vi "Untitled 0.vi"() -> ()   [LabVIEW 2016]
uses:
  <vilib>/picture/picture.llb/Draw True-Color Pixmap.vi
  <vilib>/Analysis/Matrix/Numeric/Conversions/Array To Matrix - RA2.vi
  <vilib>/imath/engines/lvmath2/RunTimeEngine/Managers/WorkSpace/UID Generator.vi
  <vilib>/Analysis/Matrix/Numeric/Conversions/Matrix To Array - RM.vi
  <vilib>/imath/engines/lvmath2/RunTimeEngine/BuiltInFunctions/rotate90/NIMS_rotate90.vi
  <instcachedir>/0/NIMS_rotate90_7DC1660D109944E092D2EB6E3185A1B6.lvgen/NIMS_rotate90_7DC1660D109944E092D2EB6E3185A1B6_004.vi
  <vilib>/imath/engines/lvmath2/RunTimeEngine/RunTimeType/NIMS_RunTimeType_From StrictType (excl LVString).vi
  <instcachedir>/0/NIMS_RunTimeType_From StrictType (excl LVString)_BBF44FB49F834B71AF7A14CCEDF8BECD.lvgen/NIMS_RunTimeType_From StrictType (excl LVString)_BBF44FB49F834B71AF7A14CCEDF8BECD_000.vi
  <vilib>/imath/engines/lvmath2/RunTimeEngine/LocalVariableDefStatement/MC_LocalVariableDefStatement_Display.vi
  <vilib>/imath/engines/lvmath2/RunTimeEngine/RangeToken/NIMS_Range_R2 - Integer.vi
  <instcachedir>/0/NIMS_Range_R2 - Integer_89B873E74E6E489885E44F751DD9C6BF.lvgen/NIMS_Range_R2 - Integer_89B873E74E6E489885E44F751DD9C6BF_000.vi
  <vilib>/imath/engines/lvmath2/RunTimeEngine/CommandStatement/MC_CommandStatement_break.vi
  <vilib>/imath/engines/lvmath2/RunTimeEngine/RangeToken/NIMS_Range.vi
  <instcachedir>/0/NIMS_Range_A7C094595B484CA7AF10685B02D808ED.lvgen/NIMS_Range_A7C094595B484CA7AF10685B02D808ED_000.vi
  <vilib>/imath/engines/lvmath2/RunTimeSupport/NIMS_Error if Not Equal.vi
  <instcachedir>/0/NIMS_Error if Not Equal_43252A79AD05436189442EC0C5E5AB8A.lvgen/NIMS_Error if Not Equal_43252A79AD05436189442EC0C5E5AB8A_001.vi
  <vilib>/imath/engines/lvmath2/RunTimeEngine/IndexRead/NIMS M(V,S).vi
  <instcachedir>/0/NIMS M(V,S)_4A7282EC9BD94252BB5D44AC841A97D6.lvgen/NIMS M(V,S)_4A7282EC9BD94252BB5D44AC841A97D6_001.vi
  <vilib>/imath/engines/lvmath2/RunTimeEngine/IndexReplace/NIMS M(V,S)=V.vi
  <instcachedir>/0/NIMS M(V,S)=V_F75C9F1BFECF4A57AE59A9C096BE65FD.lvgen/NIMS M(V,S)=V_F75C9F1BFECF4A57AE59A9C096BE65FD_001.vi
  <vilib>/imath/engines/lvmath2/RunTimeEngine/ErrorHandling/NIMS_Create Error From Enums.vi
  <vilib>/imath/engines/lvmath2/RunTimeEngine/Managers/SymbolTable/Clear UID.vi
  <vilib>/imath/engines/lvmath2/RunTimeEngine/NodeEndStatement/NIMS_NodeEndStatement_Output.vi
  <instcachedir>/0/NIMS_NodeEndStatement_Output_53EC0D466D134D7ABD903AC30B43404B.lvgen/NIMS_NodeEndStatement_Output_53EC0D466D134D7ABD903AC30B43404B_002.vi
  <vilib>/imath/engines/lvmath2/RunTimeEngine/ErrorHandling/NIMS_Finalize Error.vi
  <vilib>/imath/engines/lvmath2/RunTimeEngine/IndexRead/NIMS M(S,V).vi
  <instcachedir>/0/NIMS M(S,V)_5C1965D37F59432CA0E9661793EAFE90.lvgen/NIMS M(S,V)_5C1965D37F59432CA0E9661793EAFE90_001.vi
  <vilib>/imath/engines/lvmath2/RunTimeEngine/IndexReplace/NIMS M(S,V)=V.vi
  <instcachedir>/0/NIMS M(S,V)=V_00A569AEF20C4D858392F22F057607EC.lvgen/NIMS M(S,V)=V_00A569AEF20C4D858392F22F057607EC_001.vi
  <vilib>/imath/engines/lvmath2/RunTimeEngine/BuiltInFunctions/round/NIMS_round(DBL-S).vi
  <vilib>/imath/engines/lvmath2/RunTimeEngine/BuiltInFunctions/zeros/NIMS_M=zeros(I32,I32).vi
  <vilib>/imathl/engines/lvmath/Functions/Error Handling/Create Error.vi
  <vilib>/imath/engines/lvmath2/RunTimeEngine/RangeToken/NIMS_Range_R2 - Float.vi
  <instcachedir>/0/NIMS_Range_R2 - Float_590A1087448447AEB7F770FC082D3801.lvgen/NIMS_Range_R2 - Float_590A1087448447AEB7F770FC082D3801_000.vi
  <instcachedir>/0/NIMS_Error if Not Equal_43252A79AD05436189442EC0C5E5AB8A.lvgen/NIMS_Error if Not Equal_43252A79AD05436189442EC0C5E5AB8A_000.vi
  <vilib>/imath/engines/lvmath2/RunTimeEngine/IndexRead/NIMS M(S,$).vi
  <instcachedir>/0/NIMS M(S,$)_F24F360562DE41D8BE234322A2E15C65.lvgen/NIMS M(S,$)_F24F360562DE41D8BE234322A2E15C65_002.vi
  <vilib>/imath/engines/lvmath2/RunTimeEngine/IndexReplace/NIMS M(S,$)=V.vi
  <instcachedir>/0/NIMS M(S,$)=V_BCCFA522A894489B8FA760383D74A164.lvgen/NIMS M(S,$)=V_BCCFA522A894489B8FA760383D74A164_001.vi
  <vilib>/imath/engines/lvmath2/RunTimeEngine/IndexRead/NIMS M($,S).vi
  <instcachedir>/0/NIMS M($,S)_3E5749BBB62E49528D4765A77F1F6D98.lvgen/NIMS M($,S)_3E5749BBB62E49528D4765A77F1F6D98_002.vi
  <vilib>/imath/engines/lvmath2/RunTimeEngine/IndexReplace/NIMS M($,S)=V.vi
  <instcachedir>/0/NIMS M($,S)=V_EEA74323A7E5479BB387BE0F93352290.lvgen/NIMS M($,S)=V_EEA74323A7E5479BB387BE0F93352290_002.vi
  <instcachedir>/0/NIMS_NodeEndStatement_Output_53EC0D466D134D7ABD903AC30B43404B.lvgen/NIMS_NodeEndStatement_Output_53EC0D466D134D7ABD903AC30B43404B_010.vi
  <vilib>/imath/engines/lvmath2/RunTimeEngine/BuiltInFunctions/rand/NIMS_rand(I32,I32).vi
  <vilib>/imath/engines/lvmath2/RunTimeEngine/ErrorHandling/NIMS_Error From Error Code.vi
  <vilib>/imath/engines/lvmath2/RunTimeEngine/ArithmeticOperatorToken/NIMS_ArithmeticOperator_minus.vi
  <instcachedir>/0/NIMS_ArithmeticOperator_minus_E3B65B1D26A44BB184AFDC5B3F458E3D.lvgen/NIMS_ArithmeticOperator_minus_E3B65B1D26A44BB184AFDC5B3F458E3D_003.vi
  <instcachedir>/0/NIMS M(S,$)=V_BCCFA522A894489B8FA760383D74A164.lvgen/NIMS M(S,$)=V_BCCFA522A894489B8FA760383D74A164_000.vi
  <vilib>/imath/engines/lvmath2/RunTimeEngine/ArithmeticOperatorToken/NIMS_ArithmeticOperator_plus.vi
  <instcachedir>/0/NIMS_ArithmeticOperator_plus_0120E0498A0F4B4B9BDCAC2554767A4E.lvgen/NIMS_ArithmeticOperator_plus_0120E0498A0F4B4B9BDCAC2554767A4E_004.vi
  <instcachedir>/0/NIMS M($,S)=V_EEA74323A7E5479BB387BE0F93352290.lvgen/NIMS M($,S)=V_EEA74323A7E5479BB387BE0F93352290_001.vi
  <instcachedir>/0/NIMS_ArithmeticOperator_plus_0120E0498A0F4B4B9BDCAC2554767A4E.lvgen/NIMS_ArithmeticOperator_plus_0120E0498A0F4B4B9BDCAC2554767A4E_003.vi
  <vilib>/Analysis/Matrix/NI_Matrix.lvlib
  <vilib>/imath/engines/lvmath2/RunTimeEngine/Managers/SymbolTable/NIMS_WorkSpace.lvlib
panel:
  in  "Cluster":T1 {"y 2" scale=0.0..4.0; "Meter" scale=-360.0..360.0 scale format="%#_3g"; "y" scale=-500.0..500.0; "x" scale=-500.0..500.0}
  out "new picture 2":picture
  in  "Enum":T2(ring)
  out "new picture":picture
  in  "File Path Control":path
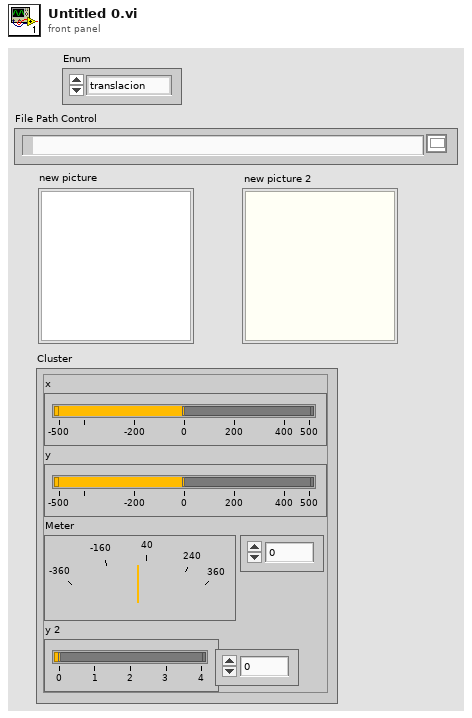
[diagram p1: front panel]
types:
  T1 = cluster{"x":dbl, "y":dbl, "Meter":dbl, "y 2":i64}
  T2 = enum16{"translacion", "giro", "extraccion", "zoom", "giroH", "giroV"}
  T3 = typedef "imagedata.ctl" = cluster{"image type":i32, "image depth":i32, "image":u8[], "mask":u8[], "colors":u32[], "Rectangle":cluster{"left":i16, "top":i16, "right":i16, "bottom":i16}}
  T4 = cluster{"left":i16, "top":i16, "right":i16, "bottom":i16}
  T5 = typedef "NI_Matrix.lvlib/RealMatrix.ctl" = dbl[][]
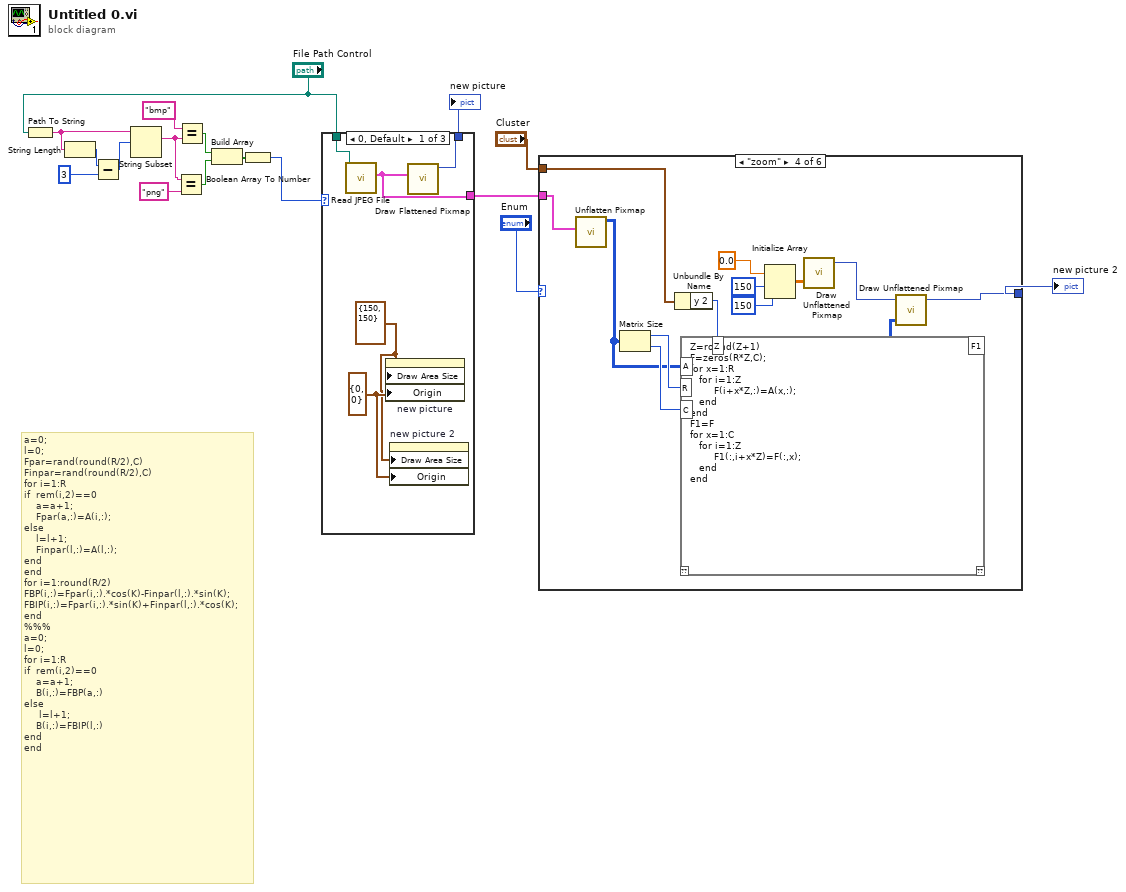
[diagram p0: block diagram]
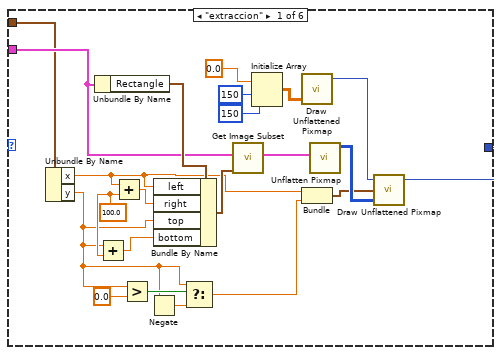
[diagram p2: hidden frame]
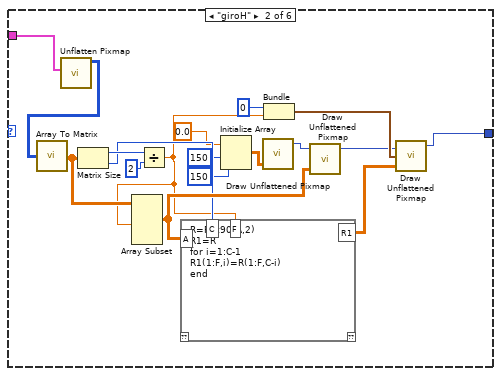
[diagram p3: hidden frame]
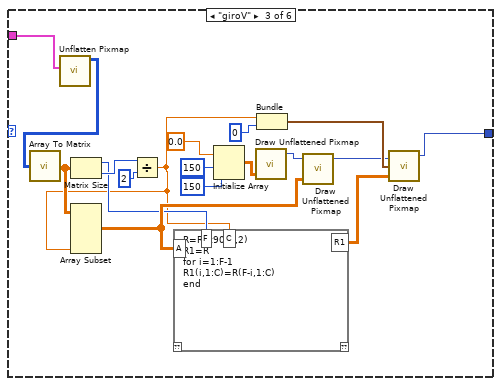
[diagram p4: hidden frame]
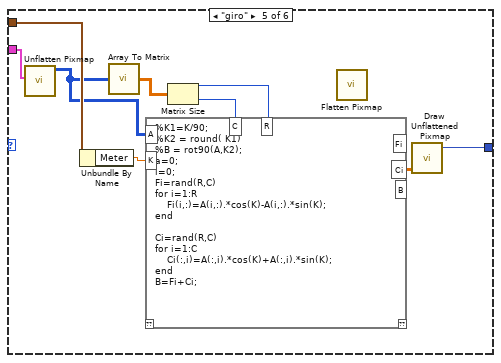
[diagram p5: hidden frame]
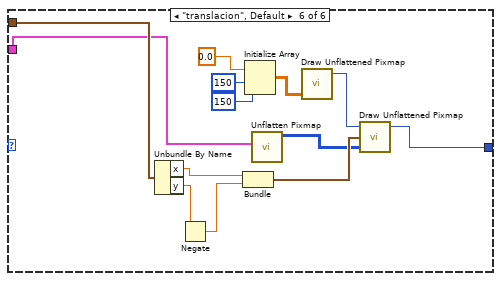
[diagram p6: hidden frame]
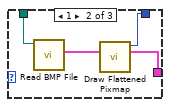
[diagram p7: hidden frame]
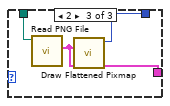
[diagram p8: hidden frame]
diagram:
  # "a=0;\nl=0;\nFpar=rand(round(R/2),C)\nFinpar=rand(round(R/2),C)\nfor i=1:R\nif  rem(i,2)==0\n    a=a+1;\n    Fpar(a,:)=A(i,:);\nelse\n    l=l+1;\n    Finpar(l,:)=A(l,:);\nend\nend\nfor i=1:round(R/2)\nFBP(i,:)=Fpar(i,:).*cos(K)-Finpar(l,:).*sin(K);\nFBIP(i,:)=Fpar(i,:).*sin(K)+Finpar(l,:).*cos(K);\nend\n%%%\na=0;\nl=0;\nfor i=1:R\nif  rem(i,2)==0\n    a=a+1;\n    B(i,:)=FBP(a,:)\nelse\n     l=l+1;\n    B(i,:)=FBIP(l,:)\nend \nend"
  n1 = Path To String(path="File Path Control") -> (string=w4:string)
  n2 = String Length(string=w4) -> (length=w17:i32)
  n3 = Subtract(x=w17, y=3) -> (x-y=w15:i32)
  n4 = String Subset(string=w4, offset (0)=w15) -> (substring=w5:string)  [unwired: 1 in]
  n5 = Equal?(x=w5, y="png" ("x")) -> (x = y?=w10:bool)
  n6 = Equal?(x="bmp", y=w5) -> (x = y?=w9:bool)
  n7 = Build Array(w9, w10) -> (w11:bool[])
  n8 = Boolean Array To Number(Boolean array=w11) -> (number=w12:u32)
  n9 = case shown="0, Default" w12 {
    tunnel: [w22 w25 w27] -> w3
    tunnel: "File Path Control" -> [w21 w24 w28]
    tunnel: [w20 w23 w26] -> w2
    frame 0, Default {
      w19 = cluster{"Horizontal":i16, "Vertical":i16} {"Horizontal"=0, "Vertical"=0} ("Origin")
      w18 = cluster{"Width":u32, "Height":u32} {"Width"=150, "Height"=150} ("Caption.Size")
      n10 = call <vilib>:"Read JPEG File.vi"("path to JPEG file"=w21) -> ("image data"=w20:T3)  [unwired: 8 in, 2 out]
      n11 = property on="new picture" class="Pict"("Draw Area Size"=w18, "Origin"=w19) -> ()  [unwired: 2 in, 2 out]
      n12 = property on="new picture 2" class="Pict"("Draw Area Size"=w18, "Origin"=w19) -> ()  [unwired: 2 in, 2 out]
      n13 = call <vilib>:"Draw Flattened Pixmap.vi"("image data"=w20) -> ("new picture"=w22:picture)  [unwired: 8 in]
    }
    frame 1 {
      n14 = call <vilib>:"Read BMP File.vi"("path to BMP file"=w24) -> ("image data"=w23:T3)  [unwired: 8 in, 2 out]
      n15 = call <vilib>:"Draw Flattened Pixmap.vi"("image data"=w23) -> ("new picture"=w25:picture)  [unwired: 8 in]
    }
    frame 2 {
      n16 = call <vilib>:"Read PNG File.vi"("path to PNG file"=w28) -> ("image data"=w26:T3)  [unwired: 8 in, 2 out]
      n17 = call <vilib>:"Draw Flattened Pixmap.vi"("image data"=w26) -> ("new picture"=w27:picture)  [unwired: 8 in]
    }
  }
  "new picture" <- w3
  n18 = case shown="\"zoom\"" "Enum" {
    tunnel: [w43 w67 w234 w394 w703 w970] -> w7
    tunnel: w2 -> [w48 w52 w219 w385 w698 w963]
    tunnel: "Cluster" -> [w42 _ _ w387 w700 w967]
    frame "extraccion" {
      w36 = 100.0 ("y")
      n19 = Unbundle By Name(w42) -> ("x"=w35:dbl, "y"=w29:dbl)
      n20 = Unbundle By Name(w48) -> ("Rectangle"=w50:T4)
      n21 = Add(x=w29, y=w36) -> (x+y=w47:dbl)
      n22 = Add(x=w35, y=w36) -> (x+y=w46:dbl)
      n23 = Greater?(x=w29, y=0.0) -> (0:w32:bool)
      n24 = Negate(x=w29) -> (-x=w30:dbl)
      n25 = Bundle By Name(cluster=w50, "left"=w35, "right"=w46, "top"=w29, "bottom"=w47) -> (w49:T4)
      n26 = Select(t=w29, s=w32, f=w30) -> (s? t:f=w31:dbl)
      n27 = call <vilib>:"Get Image Subset.vi"("subset rect"=w49, "image data"=w48) -> ("image subset"=w45:T3)  [unwired: 4 in, 1 out]
      n28 = Initialize Array(0.0 ("element"), 150 ("dimension size"), 150 ("dimension size")) -> (w38:dbl[][])
      n29 = call-poly <vilib>:"Draw Unflattened Pixmap.vi"("data (RGB format)"=w38) -> ("new picture"=w37:picture)  [unwired: 8 in]
      n30 = Bundle("x"=w35, "y"=w31) -> (w34:cluster{"x":dbl, "y":dbl})  [unwired: 1 in]
      n31 = call <vilib>:"Unflatten Pixmap.vi"("image data"=w45) -> ("24-bit pixmap"=w44:u32[][])  [unwired: 4 in, 6 out]
      n32 = call-poly <vilib>:"Draw Unflattened Pixmap.vi"("picture"=w37, "top left point(0, 0)"=w34, "data (RGB format)"=w44) -> ("new picture"=w43:picture)  [unwired: 6 in]
    }
    frame "giroH" {
      n33 = call <vilib>:"Unflatten Pixmap.vi"("image data"=w52) -> ("24-bit pixmap"=w51:u32[][])  [unwired: 4 in, 6 out]
      n34 = call-poly <vilib>:"Array To Matrix.vi"("Real 2D Array"=w51) -> ("Real Matrix"=w68:T5)
      n35 = Matrix Size(0:w68) -> (1:w61:i32, 2:w60:i32)
      n36 = Divide(x=w61, y=2) -> (x/y=w59:dbl)
      n37 = Array Subset(array=w68, length (row)=w59) -> (w63:T5)  [unwired: 3 in]
      n38 = mathscript code="R=Rot90(A,2)\nR1=R\nfor i=1:C-1\nR1(1:F,i)=R(1:F,C-i)\nend"("A"=w63, "C"=w60, "F"=w59) -> ("R1"=w58:dbl[][])  [unwired: 1 in, 1 out]
      n39 = Initialize Array(0.0 ("element"), 150 ("dimension size"), 150 ("dimension size")) -> (w54:dbl[][])
      n40 = call-poly <vilib>:"Draw Unflattened Pixmap.vi"("data (RGB format)"=w54) -> ("new picture"=w53:picture)  [unwired: 8 in]
      n41 = Bundle("y"=0, w59) -> (w64:cluster{"y":i32, dbl})  [unwired: 1 in]
      n42 = call-poly <vilib>:"Draw Unflattened Pixmap.vi"("picture"=w53, "data (RGB format)"=w63) -> ("new picture"=w62:picture)  [unwired: 7 in]
      n43 = call-poly <vilib>:"Draw Unflattened Pixmap.vi"("picture"=w62, "top left point(0, 0)"=w64, "data (RGB format)"=w58) -> ("new picture"=w67:picture)  [unwired: 6 in]
    }
    frame "giroV" {
      n44 = call <vilib>:"Unflatten Pixmap.vi"("image data"=w219) -> ("24-bit pixmap"=w218:u32[][])  [unwired: 4 in, 6 out]
      n45 = call-poly <vilib>:"Array To Matrix.vi"("Real 2D Array"=w218) -> ("Real Matrix"=w235:T5)
      n46 = Matrix Size(0:w235) -> (1:w222:i32, 2:w223:i32)
      n47 = Divide(x=w223, y=2) -> (x/y=w220:dbl)
      n48 = Array Subset(array=w235, length (col)=w220) -> (w231:T5)  [unwired: 3 in]
      n49 = mathscript code="R=Rot90(A,2)\nR1=R\nfor i=1:F-1\nR1(i,1:C)=R(F-i,1:C)\nend"("A"=w231, "F"=w222, "C"=w220) -> ("R1"=w229:dbl[][])  [unwired: 1 in, 1 out]
      n50 = Initialize Array(0.0 ("element"), 150 ("dimension size"), 150 ("dimension size")) -> (w225:dbl[][])
      n51 = call-poly <vilib>:"Draw Unflattened Pixmap.vi"("data (RGB format)"=w225) -> ("new picture"=w224:picture)  [unwired: 8 in]
      n52 = Bundle(w220, "y"=0) -> (w232:cluster{dbl, "y":i32})  [unwired: 1 in]
      n53 = call-poly <vilib>:"Draw Unflattened Pixmap.vi"("picture"=w224, "data (RGB format)"=w231) -> ("new picture"=w230:picture)  [unwired: 7 in]
      n54 = call-poly <vilib>:"Draw Unflattened Pixmap.vi"("picture"=w230, "top left point(0, 0)"=w232, "data (RGB format)"=w229) -> ("new picture"=w234:picture)  [unwired: 6 in]
    }
    frame "zoom" {
      n55 = call <vilib>:"Unflatten Pixmap.vi"("image data"=w385) -> ("24-bit pixmap"=w384:u32[][])  [unwired: 4 in, 6 out]
      n56 = Matrix Size(0:w384) -> (1:w396:i32, 2:w395:i32)
      n57 = Unbundle By Name(w387) -> ("y 2"=w386:i64)
      n58 = mathscript code="Z=round(Z+1)\nF=zeros(R*Z,C);\nfor x=1:R\n   for i=1:Z\n        F(i+x*Z,:)=A(x,:);\n   end\nend\nF1=F\nfor x=1:C\n   for i=1:Z\n        F1(:,i+x*Z)=F(:,x);\n   end\nend"("R"=w396, "C"=w395, "Z"=w386, "A"=w384) -> ("F1"=w388:u32[][])  [unwired: 1 in, 1 out]
      n59 = Initialize Array(0.0 ("element"), 150 ("dimension size"), 150 ("dimension size")) -> (w390:dbl[][])
      n60 = call-poly <vilib>:"Draw Unflattened Pixmap.vi"("data (RGB format)"=w390) -> ("new picture"=w389:picture)  [unwired: 8 in]
      n61 = call-poly <vilib>:"Draw Unflattened Pixmap.vi"("picture"=w389, "data (RGB format)"=w388) -> ("new picture"=w394:picture)  [unwired: 7 in]
    }
    frame "giro" {
      n62 = call <vilib>:"Unflatten Pixmap.vi"("image data"=w698) -> ("24-bit pixmap"=w697:u32[][])  [unwired: 4 in, 6 out]
      n63 = Unbundle By Name(w700) -> ("Meter"=w699:dbl)
      n64 = call-poly <vilib>:"Array To Matrix.vi"("Real 2D Array"=w697) -> ("Real Matrix"=w702:T5)
      n65 = Matrix Size(0:w702) -> (1:w705:i32, 2:w704:i32)
      n66 = mathscript code="%K1=K/90;\n%K2 = round( K1)\n%B = rot90(A,K2);\na=0;\nl=0;\nFi=rand(R,C)\nfor i=1:R\n    Fi(i,:)=A(i,:).*cos(K)-A(i,:).*sin(K);\nend\n\nCi=rand(R,C)\nfor i=1:C\n    Ci(:,i)=A(:,i).*cos(K)+A(:,i).*sin(K);\nend\nB=Fi+Ci;"("A"=w697, "K"=w699, "C"=w704, "R"=w705) -> ("Ci"=w701:dbl[][])  [unwired: 1 in, 3 out]
      n67 = call <vilib>:"Flatten Pixmap.vi"() -> ()  [unwired: 11 in, 1 out]
      n68 = call-poly <vilib>:"Draw Unflattened Pixmap.vi"("data (RGB format)"=w701) -> ("new picture"=w703:picture)  [unwired: 8 in]
    }
    frame "translacion", Default {
      n69 = Unbundle By Name(w967) -> ("x"=w966:dbl, "y"=w965:dbl)
      n70 = Negate(x=w965) -> (-x=w974:dbl)
      n71 = Bundle("x"=w966, w974) -> (w964:cluster{"x":dbl, dbl})  [unwired: 1 in]
      n72 = Initialize Array(0.0 ("element"), 150 ("dimension size"), 150 ("dimension size")) -> (w969:dbl[][])
      n73 = call <vilib>:"Unflatten Pixmap.vi"("image data"=w963) -> ("24-bit pixmap"=w962:u32[][])  [unwired: 4 in, 6 out]
      n74 = call-poly <vilib>:"Draw Unflattened Pixmap.vi"("data (RGB format)"=w969) -> ("new picture"=w968:picture)  [unwired: 8 in]
      n75 = call-poly <vilib>:"Draw Unflattened Pixmap.vi"("picture"=w968, "top left point(0, 0)"=w964, "data (RGB format)"=w962) -> ("new picture"=w970:picture)  [unwired: 6 in]
    }
  }
  "new picture 2" <- w7
